vi "Check Device Status.vi"(8 "error in":errorcluster, 11 "AC Comm in":refnum<class "AlicatCommBank.lvclass">) -> (0 "error out":errorcluster, 3 "AC Comm out":refnum<class "AlicatCommBank.lvclass">)   [LabVIEW 2015, in "Alicat.lvlib" / "AlicatCommBank.lvclass"]
doc: "Checks Alicat communication to determine whether all devices are present or not. If not, the device is removed and a warning will tell the user which device(s) were removed."
uses:
  AlicatCommBank.lvclass
  AlicatCommBank.lvclass/AlicatCommBank.ctl
  Reusable/Serial IO/Serial IO.lvclass/Serial IO.ctl
  Reusable/Serial IO/Write present.vi
  Alicat.lvclass
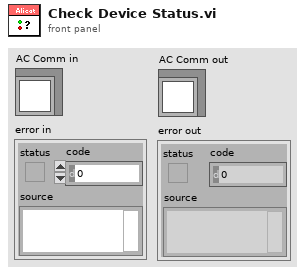
[diagram p1: front panel]
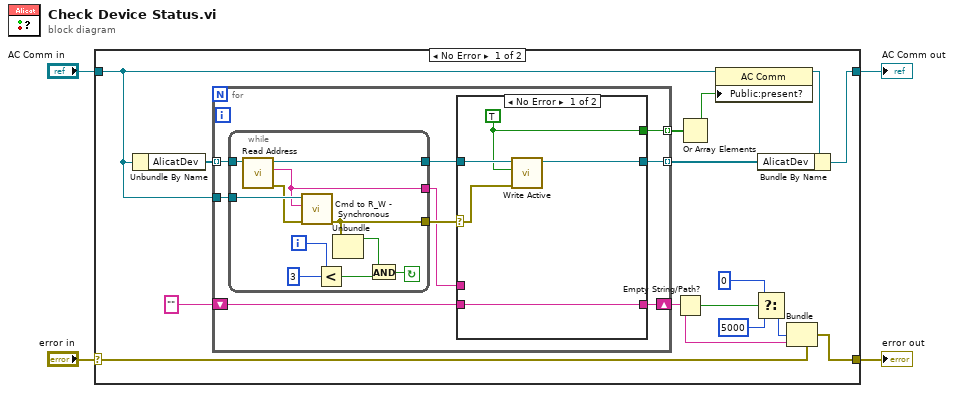
[diagram p0: block diagram]
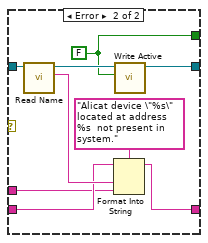
[diagram p2: hidden frame]
diagram:
  n1 = case shown="No Error" "error in" {
    selector: "error in" -> [w16 w55]
    tunnel: [w10 w55] -> w3
    tunnel: [w18 w54] -> w1
    tunnel: "AC Comm in" -> [w8 w54]
    frame No Error {
      n2 = Unbundle By Name(w8) -> ("AlicatDev"=w19:refnum<class "Alicat.lvclass">[])
      n3 = for {
        tunnel: w19 -> [w24] mode=indexing
        tunnel: w8 -> [w28]
        shift-right: [w25] -> w12
        shift-left: "" -> [w26]
        tunnel: [w21] -> w9 mode=indexing
        tunnel: [w20] -> w6 mode=indexing
        n4 = while {
          tunnel: w28 -> [w39]
          tunnel: [w34] -> w27
          tunnel: w24 -> [w38]
          tunnel: [w37] -> w23
          tunnel: [w36] -> w22
          i -> [w30]
          stop <- w33 continue-if-true
          n5 = call "Read Address.vi"("Alicat in"=w38) -> ("error out"=w35:errorcluster, "Address"=w36:string, "Alicat out"=w37:refnum<class "Alicat.lvclass">)  [unwired: 8 in]
          n6 = call-dynamic "Cmd to R_W - Synchronous.vi"("error in"=w35, "write buffer"=w36, "Serial IO in"=w39) -> ("error out"=w34:errorcluster)  [unwired: 6 in, 2 out]
          n7 = Less?(x=w30, y=3) -> (x < y?=w31:bool)
          n8 = Unbundle(w34) -> ("status"=w32:bool)  [unwired: 2 out]
          n9 = And(x=w32, y=w31) -> (x .and. y?=w33:bool)
        }
        n10 = case shown="No Error" w27 {
          selector: w27 -> [w41 _]
          tunnel: w23 -> [w43 w53]
          tunnel: w26 -> [w44 w50]
          tunnel: [w44 w49] -> w25
          tunnel: w22 -> [_ w48]
          tunnel: [w42 w46] -> w21
          tunnel: [w40 w45] -> w20
          frame No Error {
            w40 = TRUE ("Active?")
            n11 = call "Write Active.vi"("error in"=w41, "Active?"=w40, "Alicat in"=w43) -> ("Alicat out"=w42:refnum<class "Alicat.lvclass">)  [unwired: 7 in, 1 out]
          }
          frame Error {
            w45 = FALSE ("Active?")
            n12 = call "Read Name.vi"("Alicat in"=w53) -> ("Name"=w51:string, "Alicat out"=w47:refnum<class "Alicat.lvclass">)  [unwired: 8 in, 1 out]
            n13 = Format Into String(format string="Alicat device \"%s\" located at address %s  not present in system." ("initial string"), initial string=w50, w51, w48) -> (resulting string=w49:string)  [unwired: 1 in, 1 out]
            n14 = call "Write Active.vi"("Active?"=w45, "Alicat in"=w47) -> ("Alicat out"=w46:refnum<class "Alicat.lvclass">)  [unwired: 8 in, 1 out]
          }
        }
      }
      n15 = Empty String/Path?(string/path=w12) -> (empty?=w15:bool)
      n16 = Or Array Elements(Boolean array=w6) -> (logical OR=w5:bool)
      n17 = property class="AC Comm"(reference=w8, "Public:present?"=w5) -> (reference out=w7:refnum<class "AlicatCommBank.lvclass">)  [unwired: 1 in, 1 out]
      n18 = Select(t=0 ("code"), s=w15, f=5000 ("code")) -> (s? t:f=w11:i32)
      n19 = Bundle By Name(cluster=w7, "AlicatDev"=w9) -> (w18:refnum<class "AlicatCommBank.lvclass">)
      n20 = Bundle(cluster=w16, "code"=w11, "source"=w12) -> (w10:errorcluster)  [unwired: 1 in]
    }
    frame Error {
    }
  }
  "error out" <- w3
  "AC Comm out" <- w1
